vi "Continuous acquisition.vi"() -> ()   [LabVIEW 2024]
uses:
  <instrlib>/niScope/Configure/Trigger/niScope Configure Trigger Edge.vi
  <instrlib>/niScope/Acquire/niScope Multi Read Cluster.vi
panel:
  in  "Triggering:Trigger Modifier":i32(ring)=1 items=["None"=1, "Auto Trigger"=2]
  out "specific error cleared?":bool
  in  "Vertical Range (V)":dbl=5.0 format="%_3g"
  in  "Stop":bool
  in  "Resource Name":refnum<k15>="Dev1" caption="Resource Name(s)"
  in  "Input Impedance":u32(ring)=2 items=["1 mega ohm"=0, "50 ohms"=2]
  in  "Trigger Level (V)":dbl=0.5 caption="Trigger Level" format="%.2f"
  in  "Vertical Coupling":i32(ring)=1 items=["AC", "DC", "Ground"]
  in  "Min Record Length":i32=40000
  in  "Min. Sample Rate":dbl=10000000.0 format="%#_6p"
  out "Waveform From Scope":T1(graph) caption="Waveform from Scope"
  in  "Channel(s)":string="0"
  # "Vertical"
  # "Horizontal"
  # "Triggering"
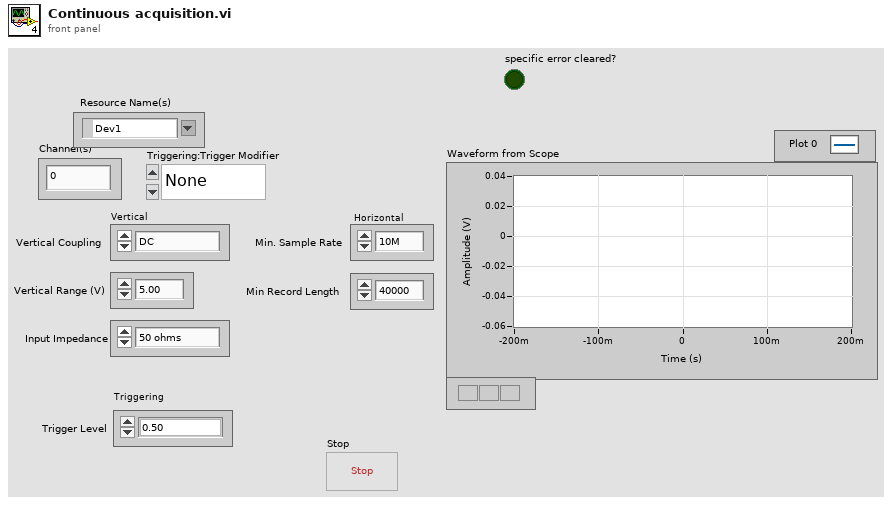
[diagram p1: front panel]
types:
  T1 = cluster{"relativeInitialX":dbl, "xIncrement":dbl, "wfm":dbl[]}[]
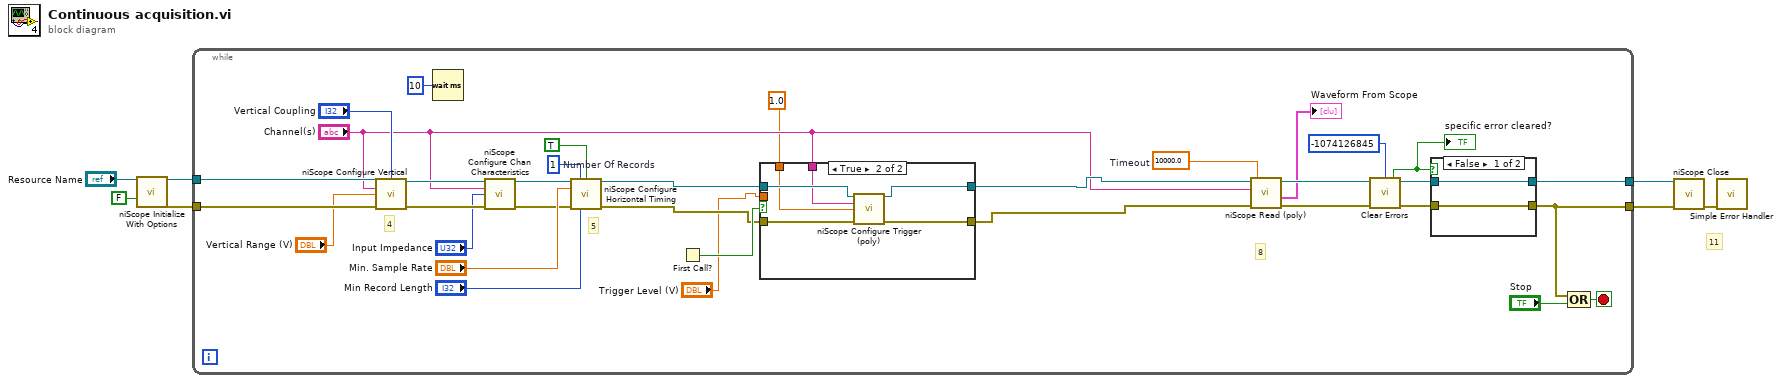
[diagram p0: block diagram]
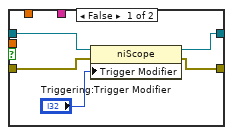
[diagram p2: hidden frame]
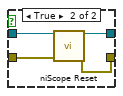
[diagram p3: hidden frame]
diagram:
  # "11"
  n1 = call <instrlib>:"niScope Initialize With Options.vi"("resource name"="Resource Name", "reset device"=FALSE) -> ("instrument handle"=w6:refnum<k15>, "error out"=w5:errorcluster)  [unwired: 12 in]
  n2 = while {
    tunnel: w6 -> [w29]
    tunnel: w5 -> [w28]
    tunnel: [w18] -> w3
    tunnel: [w19] -> w2
    stop <- w26 stop-if-true
    w31 = 1  # Number Of Records
    w37 = 10000.0  # Timeout
    # "8"
    # "5"
    # "4"
    n3 = call <instrlib>:"niScope Configure Vertical.vi"("instrument handle"=w29, "vertical coupling"="Vertical Coupling", "channels"="Channel(s)", "vertical range"="Vertical Range (V)", "error in"=w28) -> ("instrument handle out"=w35:refnum<k15>, "error out"=w36:errorcluster)  [unwired: 9 in]
    n4 = Wait (ms)(milliseconds to wait=u32 10 ("Millisecond Multiple")) -> ()  [unwired: 1 out]
    n5 = call <instrlib>:"niScope Configure Chan Characteristics.vi"("instrument handle"=w35, "channels"="Channel(s)", "input impedance"="Input Impedance", "error in"=w36) -> ("instrument handle out"=w34:refnum<k15>, "error out"=w33:errorcluster)  [unwired: 10 in]
    n6 = call <instrlib>:"niScope Configure Horizontal Timing.vi"("instrument handle"=w34, "number of records"=w31, "enforce realtime"=TRUE ("Enforce Realtime"), "min sample rate"="Min. Sample Rate", "error in"=w33, "min record length"="Min Record Length") -> ("instrument handle out"=w15:refnum<k15>, "error out"=w14:errorcluster)  [unwired: 8 in]
    n7 = First Call?() -> (First Call?: T/F=w16:bool)
    n8 = case shown="True" w16 {
      tunnel: w15 -> [w44 w51]
      tunnel: w14 -> [w43 w50]
      tunnel: "Trigger Level (V)" -> [_ _]
      tunnel: [w45 w49] -> w12
      tunnel: [w42 w48] -> w11
      tunnel: "Channel(s)" -> [_ w47]
      tunnel: 1.0 ("trigger level") -> [_ w46]
      frame False {
        n9 = property class="niScope"(reference=w44, error in=w43, "Trigger Modifier"="Triggering:Trigger Modifier") -> (reference out=w45:refnum<k15>, error out=w42:errorcluster)
      }
      frame True {
        n10 = call-poly <instrlib>:"niScope Configure Trigger (poly).vi"("instrument handle"=w51, "trigger source"=w47, "trigger level"=w46, "error in"=w50) -> ("instrument handle out"=w49:refnum<k15>, "error out"=w48:errorcluster)  [unwired: 10 in]
      }
    }
    n11 = call-poly <instrlib>:"niScope Read (poly).vi"("timeout"=w37, "error in"=w11, "channels"="Channel(s)", "instrument handle"=w12) -> ("error out"=w25:errorcluster, "waveform"=→"Waveform From Scope":T1, "instrument handle out"=w21:refnum<k15>)  [unwired: 4 in, 1 out]
    n12 = call <vilib>:"Clear Errors.vi"("error in (no error)"=w25, "specific error code to clear (0: all)"=-1074126845) -> ("error out"=w20:errorcluster, "specific error cleared?"=w17:bool)  [unwired: 4 in]
    "specific error cleared?" <- w17
    n13 = case shown="False" w17 {
      tunnel: w21 -> [w53 w57]
      tunnel: w20 -> [w52 w56]
      tunnel: [w52 w55] -> w19
      tunnel: [w53 w54] -> w18
      frame False {
      }
      frame True {
        n14 = call <instrlib>:"niScope Reset.vi"("instrument handle"=w57, "error in"=w56) -> ("instrument handle out"=w54:refnum<k15>, "error out"=w55:errorcluster)  [unwired: 12 in]
      }
    }
    n15 = Compound Arithmetic op=OR(w19, "Stop") -> (w26:bool)
  }
  n16 = call <instrlib>:"niScope Close.vi"("instrument handle"=w3, "error in"=w2) -> ("error out"=w4:errorcluster)  [unwired: 13 in]
  n17 = call <vilib>:"Simple Error Handler.vi"("error in (no error)"=w4) -> ()  [unwired: 4 in, 5 out]
